vi "Check_Particular_Condition.vi"(9 "Cluster of conditions":T1 caption="Condition" {"Specifier(s)"."Validity criteria(s)"."Validity value" min=0.0 step=0.1 format="%.2g"; "Specifier(s)"."Value" step=1.0 format="%#.2g"}, 10 "Current animal coordinates and stats":T8 {"Measurements and statistics"."Running, perc. of time" format="%05.2f"}, 11 "Frame length, ms":dbl) -> (2 "Stop check":bool, 3 "Condition is met":bool)   [LabVIEW 2018, in "TTL IO.lvlib"]
uses:
  TTL IO.lvlib
  SubVi's/Controls/CTL_Full_data_frame.ctl
  SubVi's/Controls/CTL_Animal_Coordinates_and_Speed.ctl
  SubVi's/Controls/CTL_Measurements_and_Statistics.ctl
  SubVi's/Controls/CTL_Conditions_Cluster.ctl
  SubVi's/Controls/CTL_Condition_type.ctl
  SubVi's/Controls/CTL_Comparison_type.ctl
  SubVi's/Controls/CTL_Validity_check_criteria.ctl
  SubVi's/Controls/CTL_Response_info.ctl
  SubVi's/Controls/CTL_Condition_response_type.ctl
  SubVi's/Controls/CTL_Reponse_port_info.ctl
  <vilib>/ptbypt/NI_PtbyPt.lvlib
  Common_Resources.lvlib
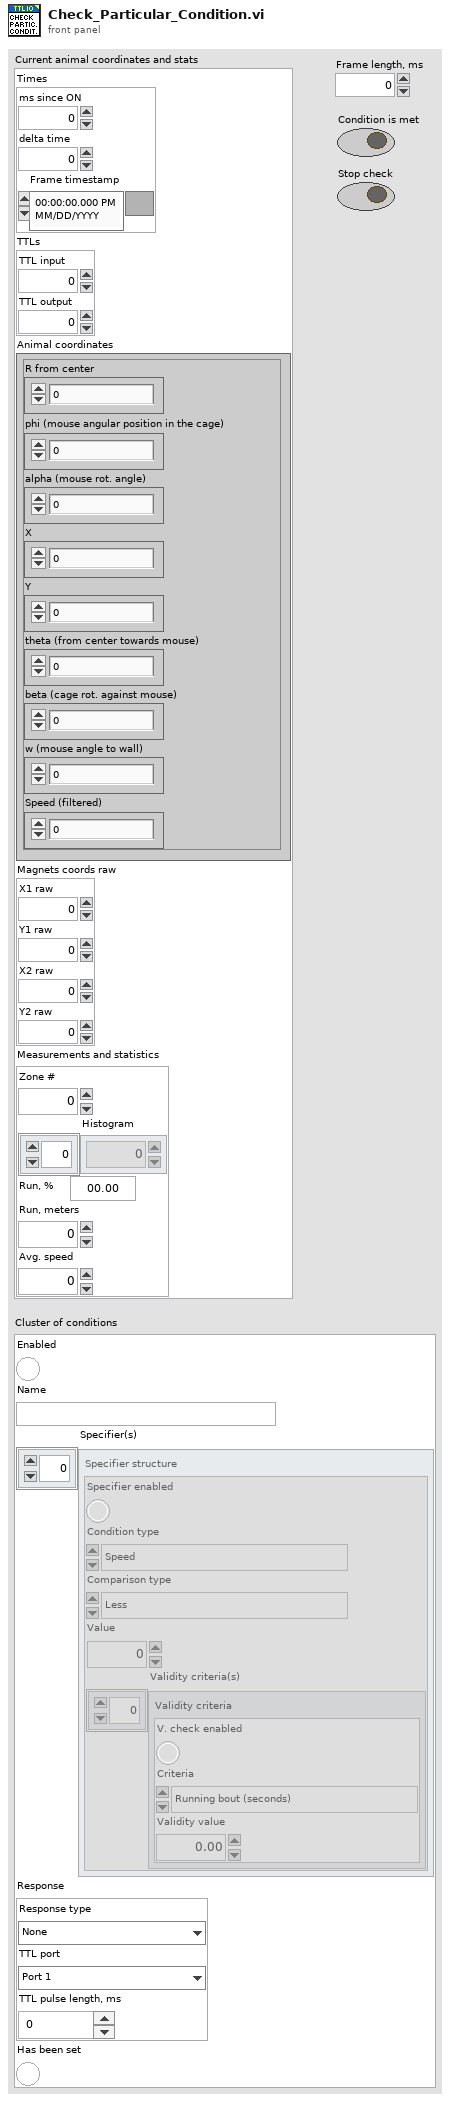
[diagram p1: front panel]
types:
  T1 = typedef "Common_Resources.lvlib/CTL_Conditions_Cluster.ctl" = cluster{"Enabled":bool, "Name":string, "Specifier(s)":cluster{"Specifier enabled":bool, "Condition type":T2, "Comparison type":T3, "Value":dbl, "Validity criteria(s)":cluster{"V. check enabled":bool, "Criteria":T4, "Validity value":dbl}[]}[], "Response":T5, "Has been set":bool}
  T2 = typedef "Common_Resources.lvlib/CTL_Condition_type.ctl" = enum16{"Speed", "Zone", "Angle to wall"}
  T3 = typedef "Common_Resources.lvlib/CTL_Comparison_type.ctl" = enum16{"Less", "Less or Equal", "Equal", "Greater or Equal", "Greater", "Not Equal"}
  T4 = typedef "Common_Resources.lvlib/CTL_Validity_check_criteria.ctl" = enum16{"Running bout (seconds)", "Running bout (meters)"}
  T5 = typedef "Common_Resources.lvlib/CTL_Response_info.ctl" = cluster{"Response type":T6, "TTL port":T7, "TTL pulse length, ms":dbl}
  T6 = typedef "Common_Resources.lvlib/CTL_Condition_response_type.ctl" = enum16{"None", "Air puff", "Liquid reward"}
  T7 = typedef "Common_Resources.lvlib/CTL_Reponse_port_info.ctl" = enum16{"Port 1", "Port 2", "Port 3", "Port 4"}
  T8 = typedef "Common_Resources.lvlib/CTL_Full_data_frame.ctl" = cluster{"Times":cluster{"ms since ON":u32, "delta time":u32, "Frame timestamp":timestamp}, "TTLs":cluster{"TTL input":i16, "TTL output":i16}, "Animal coordinates":T9, "Magnets coords raw":cluster{"X1 raw":dbl, "Y1 raw":dbl, "X2 raw":dbl, "Y2 raw":dbl}, "Measurements and statistics":T10}
  T9 = typedef "Common_Resources.lvlib/CTL_Animal_Coordinates_and_Speed.ctl" = cluster{"R from center":dbl, "phi (mouse angular position in the cage)":dbl, "alpha (mouse rot. angle)":dbl, "X":dbl, "Y":dbl, "theta (from center towards mouse)":dbl, "beta (cage rot. against mouse)":dbl, "w (mouse angle to wall)":dbl, "Speed (filtered)":dbl}
  T10 = typedef "Common_Resources.lvlib/CTL_Measurements_and_Statistics.ctl" = cluster{"Zone #":i8, "Histogram":dbl[], "Running, perc. of time":dbl, "Run, meters":dbl, "Avg. speed":dbl}
  T11 = cluster{"Specifier enabled":bool, "Condition type":T2, "Comparison type":T3, "Value":dbl, "Validity criteria(s)":cluster{"V. check enabled":bool, "Criteria":T4, "Validity value":dbl}[]}[]
  T12 = cluster{"Specifier enabled":bool, "Condition type":T2, "Comparison type":T3, "Value":dbl, "Validity criteria(s)":cluster{"V. check enabled":bool, "Criteria":T4, "Validity value":dbl}[]}
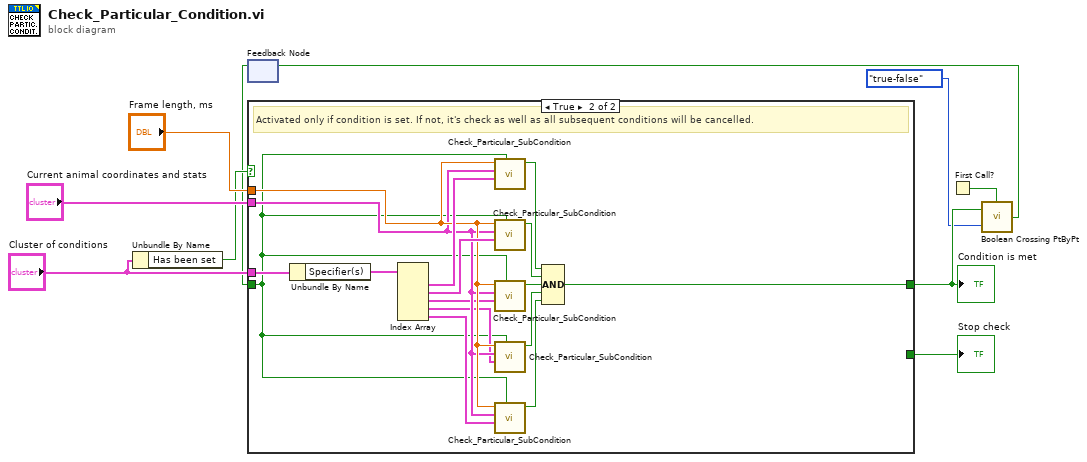
[diagram p0: block diagram]
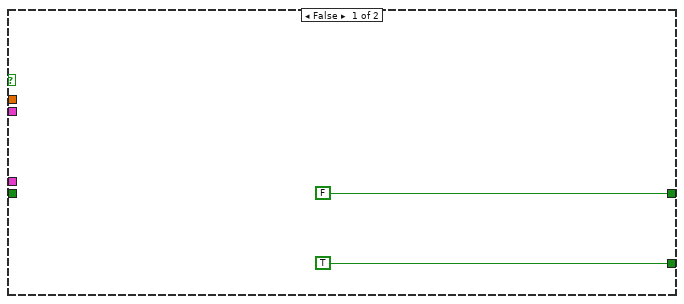
[diagram p2: hidden frame]
diagram:
  n1 = Unbundle By Name("Cluster of conditions") -> ("Has been set"=w7:bool)
  n2 = feedback #1() -> (w2:bool)  [unwired: 1 in]
  n3 = case shown="True" w7 {
    tunnel: "Cluster of conditions" -> [_ w28]
    tunnel: [TRUE _] -> w10
    tunnel: [FALSE w14] -> w5
    tunnel: "Current animal coordinates and stats" -> [_ w23]
    tunnel: "Frame length, ms" -> [_ w24]
    tunnel: w2 -> [_ w13]
    frame False {
    }
    frame True {
      # "Activated only if condition is set. If not, it's check as well as all subsequent conditions will be cancelled."
      n4 = Unbundle By Name(w28) -> ("Specifier(s)"=w27:T11)
      n5 = Index Array(array=w27) -> (element #1=w26:T12, element #2=w25:T12, element #3=w22:T12, element #4=w21:T12, element #5=w20:T12)  [unwired: 5 in]
      n6 = call "Check_Particular_SubCondition.vi"("Reset?"=w13, "Specifier structure"=w26, "Current animal coordinates and stats"=w23, "Frame length, ms"=w24) -> ("Valid?"=w19:bool)  [unwired: 7 in]
      n7 = call "Check_Particular_SubCondition.vi"("Reset?"=w13, "Specifier structure"=w25, "Current animal coordinates and stats"=w23, "Frame length, ms"=w24) -> ("Valid?"=w18:bool)  [unwired: 7 in]
      n8 = call "Check_Particular_SubCondition.vi"("Reset?"=w13, "Specifier structure"=w22, "Current animal coordinates and stats"=w23, "Frame length, ms"=w24) -> ("Valid?"=w17:bool)  [unwired: 7 in]
      n9 = call "Check_Particular_SubCondition.vi"("Reset?"=w13, "Specifier structure"=w21, "Current animal coordinates and stats"=w23, "Frame length, ms"=w24) -> ("Valid?"=w16:bool)  [unwired: 7 in]
      n10 = call "Check_Particular_SubCondition.vi"("Reset?"=w13, "Specifier structure"=w20, "Current animal coordinates and stats"=w23, "Frame length, ms"=w24) -> ("Valid?"=w15:bool)  [unwired: 7 in]
      n11 = Compound Arithmetic op=AND(w19, w18, w17, w16, w15) -> (w14:bool)
    }
  }
  "Stop check" <- w10
  "Condition is met" <- w5
  n12 = First Call?() -> (First Call?: T/F=w1:bool)
  n13 = call <vilib>:"Boolean Crossing PtByPt.vi"("initialize"=w1, "direction"=enum16{"either", "false-true", "true-false"}."true-false", "input"=w5) -> ("crossing"=w3:bool)
  n14 = feedback-in #1(w3) -> ()
